vi "dbc Initial.vi"(8 "error in (no error)":errorcluster) -> (0 "error out":errorcluster, 2 "NameShort":string[][](array[string])=[["Radar_AK_AMP", "Radar_AK_ANG", "Radar_AK_BSD_FLG", "Radar_AK_DST", "Radar_AK_ELE", "Radar_AK_EXST_PRB", "Radar_AK_Ego_Car_SPD", "Radar_AK_ID", "Radar_AK_LNG_ACC", "Radar_AK_MOV_FLG", "Radar_AK_RESERVE", "Radar_AK_SPD", "Radar_AK_Vx", "Radar_AK_Vy", "Radar_AK_Vz", "", "", "", "", "", "", "", "", "", "", "", "", "", "", ""], ["Radar_BK_2_AMP", "Radar_BK_2_ANG", "Radar_BK_2_DST", "Radar_BK_2_ELE", "Radar_BK_2_SPD", "Radar_BK_3_AMP", "Radar_BK_3_ANG", "Radar_BK_3_DST", "Radar_BK_3_ELE", "Radar_BK_3_SPD", "Radar_BK_4_AMP", "Radar_BK_4_ANG", "Radar_BK_4_DST", "Radar_BK_4_ELE", "Radar_BK_4_SPD", "Radar_BK_5_AMP", "Radar_BK_5_ANG", "Radar_BK_5_DST", "Radar_BK_5_ELE", "Radar_BK_5_SPD", "Radar_BK_6_AMP", "Radar_BK_6_ANG", "Radar_BK_6_DST", "Radar_BK_6_ELE", "Radar_BK_6_SPD", "Radar_BK_AMP", "Radar_BK_ANG", "Radar_BK_DST", "Radar_BK_ELE", "Radar_BK_SPD"], ["Radar_Header_Cdi_Number", "Radar_Header_Frame_Peroid", "Radar_Header_Frame_Type", "Radar_Header_Frame_id", "Radar_Header_Raw_Number", "Radar_Header_Track_Output_Number", "", "", "", "", "", "", "", "", "", "", "", "", "", "", "", "", "", "", "", "", "", "", "", ""], ["Radar_AK_Header_Number", "Radar_AK_Run_Time", "", "", "", "", "", "", "", "", "", "", "", "", "", "", "", "", "", "", "", "", "", "", "", "", "", "", "", ""]], 3 "Session Out":refnum<k21>[](array[refnum]), 5 "ID":u32[](array[numeric])=[1280, 1024, 768, 816] format="%.0x")   [LabVIEW 2024]
uses:
  <vilib>/xnet/xnet.llb/XNET Create Session (Conversion).vi
  <resource>/objmgr/xnet.rc
panel:
  out "Sigs":refnum<k21>[][](array[refnum])
  out "XNET_DBC":T1(array[cluster])=[[{"NameShort"="Radar_AK_AMP", "ByteOrdr"=0, "StartBit"=64, "NumBits"=16, "Max"=327.67, "Min"=-327.68, "ScaleFac"=0.01, "ScaleOff"=0.0, "Comment"="", "Unit"="dB", "PDU"="Radar2ECU_AK_FRAME_0x500_pdu\nradar com1"}, {"NameShort"="Radar_AK_ANG", "ByteOrdr"=0, "StartBit"=16, "NumBits"=16, "Max"=327.67, "Min"=-327.68, "ScaleFac"=0.01, "ScaleOff"=0.0, "Comment"="", "Unit"="deg", "PDU"="Radar2ECU_AK_FRAME_0x500_pdu\nradar com1"}, {"NameShort"="Radar_AK_BSD_FLG", "ByteOrdr"=0, "StartBit"=192, "NumBits"=1, "Max"=1.0, "Min"=0.0, "ScaleFac"=1.0, "ScaleOff"=0.0, "Comment"="", "Unit"="", "PDU"="Radar2ECU_AK_FRAME_0x500_pdu\nradar com1"}, {"NameShort"="Radar_AK_DST", "ByteOrdr"=0, "StartBit"=48, "NumBits"=16, "Max"=327.67, "Min"=-327.68, "ScaleFac"=0.01, "ScaleOff"=0.0, "Comment"="", "Unit"="m", "PDU"="Radar2ECU_AK_FRAME_0x500_pdu\nradar com1"}, {"NameShort"="Radar_AK_ELE", "ByteOrdr"=0, "StartBit"=80, "NumBits"=16, "Max"=327.67, "Min"=-327.68, "ScaleFac"=0.01, "ScaleOff"=0.0, "Comment"="", "Unit"="deg", "PDU"="Radar2ECU_AK_FRAME_0x500_pdu\nradar com1"}, {"NameShort"="Radar_AK_EXST_PRB", "ByteOrdr"=0, "StartBit"=144, "NumBits"=16, "Max"=327.67, "Min"=-327.68, "ScaleFac"=0.01, "ScaleOff"=0.0, "Comment"="", "Unit"="%", "PDU"="Radar2ECU_AK_FRAME_0x500_pdu\nradar com1"}, {"NameShort"="Radar_AK_Ego_Car_SPD", "ByteOrdr"=0, "StartBit"=176, "NumBits"=16, "Max"=327.67, "Min"=-327.68, "ScaleFac"=0.01, "ScaleOff"=0.0, "Comment"="", "Unit"="m/s", "PDU"="Radar2ECU_AK_FRAME_0x500_pdu\nradar com1"}, {"NameShort"="Radar_AK_ID", "ByteOrdr"=0, "StartBit"=0, "NumBits"=16, "Max"=65535.0, "Min"=0.0, "ScaleFac"=1.0, "ScaleOff"=0.0, "Comment"="", "Unit"="", "PDU"="Radar2ECU_AK_FRAME_0x500_pdu\nradar com1"}, {"NameShort"="Radar_AK_LNG_ACC", "ByteOrdr"=0, "StartBit"=160, "NumBits"=16, "Max"=327.67, "Min"=-327.68, "ScaleFac"=0.01, "ScaleOff"=0.0, "Comment"="", "Unit"="m/s2", "PDU"="Radar2ECU_AK_FRAME_0x500_pdu\nradar com1"}, {"NameShort"="Radar_AK_MOV_FLG", "ByteOrdr"=0, "StartBit"=193, "NumBits"=1, "Max"=1.0, "Min"=0.0, "ScaleFac"=1.0, "ScaleOff"=0.0, "Comment"="", "Unit"="", "PDU"="Radar2ECU_AK_FRAME_0x500_pdu\nradar com1"}, {"NameShort"="Radar_AK_RESERVE", "ByteOrdr"=0, "StartBit"=194, "NumBits"=6, "Max"=63.0, "Min"=0.0, "ScaleFac"=1.0, "ScaleOff"=0.0, "Comment"="", "Unit"="", "PDU"="Radar2ECU_AK_FRAME_0x500_pdu\nradar com1"}, {"NameShort"="Radar_AK_SPD", "ByteOrdr"=0, "StartBit"=32, "NumBits"=16, "Max"=327.67, "Min"=-327.68, "ScaleFac"=0.01, "ScaleOff"=0.0, "Comment"="", "Unit"="m/s", "PDU"="Radar2ECU_AK_FRAME_0x500_pdu\nradar com1"}, {"NameShort"="Radar_AK_Vx", "ByteOrdr"=0, "StartBit"=96, "NumBits"=16, "Max"=0.0, "Min"=0.0, "ScaleFac"=0.01, "ScaleOff"=0.0, "Comment"="", "Unit"="", "PDU"="Radar2ECU_AK_FRAME_0x500_pdu\nradar com1"}, {"NameShort"="Radar_AK_Vy", "ByteOrdr"=0, "StartBit"=112, "NumBits"=16, "Max"=0.0, "Min"=0.0, "ScaleFac"=0.01, "ScaleOff"=0.0, "Comment"="", "Unit"="", "PDU"="Radar2ECU_AK_FRAME_0x500_pdu\nradar com1"}, {"NameShort"="Radar_AK_Vz", "ByteOrdr"=0, "StartBit"=128, "NumBits"=16, "Max"=0.0, "Min"=0.0, "ScaleFac"=0.01, "ScaleOff"=0.0, "Comment"="", "Unit"="", "PDU"="Radar2ECU_AK_FRAME_0x500_pdu\nradar com1"}, {"NameShort"="", "ByteOrdr"=0, "StartBit"=0, "NumBits"=0, "Max"=0.0, "Min"=0.0, "ScaleFac"=0.0, "ScaleOff"=0.0, "Comment"="", "Unit"="", "PDU"=""}, {"NameShort"="", "ByteOrdr"=0, "StartBit"=0, "NumBits"=0, "Max"=0.0, "Min"=0.0, "ScaleFac"=0.0, "ScaleOff"=0.0, "Comment"="", "Unit"="", "PDU"=""}, {"NameShort"="", "ByteOrdr"=0, "StartBit"=0, "NumBits"=0, "Max"=0.0, "Min"=0.0, "ScaleFac"=0.0, "ScaleOff"=0.0, "Comment"="", "Unit"="", "PDU"=""}, {"NameShort"="", "ByteOrdr"=0, "StartBit"=0, "NumBits"=0, "Max"=0.0, "Min"=0.0, "ScaleFac"=0.0, "ScaleOff"=0.0, "Comment"="", "Unit"="", "PDU"=""}, {"NameShort"="", "ByteOrdr"=0, "StartBit"=0, "NumBits"=0, "Max"=0.0, "Min"=0.0, "ScaleFac"=0.0, "ScaleOff"=0.0, "Comment"="", "Unit"="", "PDU"=""}, {"NameShort"="", "ByteOrdr"=0, "StartBit"=0, "NumBits"=0, "Max"=0.0, "Min"=0.0, "ScaleFac"=0.0, "ScaleOff"=0.0, "Comment"="", "Unit"="", "PDU"=""}, {"NameShort"="", "ByteOrdr"=0, "StartBit"=0, "NumBits"=0, "Max"=0.0, "Min"=0.0, "ScaleFac"=0.0, "ScaleOff"=0.0, "Comment"="", "Unit"="", "PDU"=""}, {"NameShort"="", "ByteOrdr"=0, "StartBit"=0, "NumBits"=0, "Max"=0.0, "Min"=0.0, "ScaleFac"=0.0, "ScaleOff"=0.0, "Comment"="", "Unit"="", "PDU"=""}, {"NameShort"="", "ByteOrdr"=0, "StartBit"=0, "NumBits"=0, "Max"=0.0, "Min"=0.0, "ScaleFac"=0.0, "ScaleOff"=0.0, "Comment"="", "Unit"="", "PDU"=""}, {"NameShort"="", "ByteOrdr"=0, "StartBit"=0, "NumBits"=0, "Max"=0.0, "Min"=0.0, "ScaleFac"=0.0, "ScaleOff"=0.0, "Comment"="", "Unit"="", "PDU"=""}, {"NameShort"="", "ByteOrdr"=0, "StartBit"=0, "NumBits"=0, "Max"=0.0, "Min"=0.0, "ScaleFac"=0.0, "ScaleOff"=0.0, "Comment"="", "Unit"="", "PDU"=""}, {"NameShort"="", "ByteOrdr"=0, "StartBit"=0, "NumBits"=0, "Max"=0.0, "Min"=0.0, "ScaleFac"=0.0, "ScaleOff"=0.0, "Comment"="", "Unit"="", "PDU"=""}, {"NameShort"="", "ByteOrdr"=0, "StartBit"=0, "NumBits"=0, "Max"=0.0, "Min"=0.0, "ScaleFac"=0.0, "ScaleOff"=0.0, "Comment"="", "Unit"="", "PDU"=""}, {"NameShort"="", "ByteOrdr"=0, "StartBit"=0, "NumBits"=0, "Max"=0.0, "Min"=0.0, "ScaleFac"=0.0, "ScaleOff"=0.0, "Comment"="", "Unit"="", "PDU"=""}, {"NameShort"="", "ByteOrdr"=0, "StartBit"=0, "NumBits"=0, "Max"=0.0, "Min"=0.0, "ScaleFac"=0.0, "ScaleOff"=0.0, "Comment"="", "Unit"="", "PDU"=""}], [{"NameShort"="Radar_BK_2_AMP", "ByteOrdr"=0, "StartBit"=128, "NumBits"=16, "Max"=327.67, "Min"=-327.68, "ScaleFac"=0.01, "ScaleOff"=0.0, "Comment"="", "Unit"="dB", "PDU"="Radar2ECU_BK_FRAME_0x400_pdu\nradar com1"}, {"NameShort"="Radar_BK_2_ANG", "ByteOrdr"=0, "StartBit"=80, "NumBits"=16, "Max"=327.67, "Min"=-327.68, "ScaleFac"=0.01, "ScaleOff"=0.0, "Comment"="", "Unit"="deg", "PDU"="Radar2ECU_BK_FRAME_0x400_pdu\nradar com1"}, {"NameShort"="Radar_BK_2_DST", "ByteOrdr"=0, "StartBit"=112, "NumBits"=16, "Max"=327.67, "Min"=-327.68, "ScaleFac"=0.01, "ScaleOff"=0.0, "Comment"="", "Unit"="m", "PDU"="Radar2ECU_BK_FRAME_0x400_pdu\nradar com1"}, {"NameShort"="Radar_BK_2_ELE", "ByteOrdr"=0, "StartBit"=144, "NumBits"=16, "Max"=327.67, "Min"=-327.68, "ScaleFac"=0.01, "ScaleOff"=0.0, "Comment"="", "Unit"="deg", "PDU"="Radar2ECU_BK_FRAME_0x400_pdu\nradar com1"}, {"NameShort"="Radar_BK_2_SPD", "ByteOrdr"=0, "StartBit"=96, "NumBits"=16, "Max"=327.67, "Min"=-327.68, "ScaleFac"=0.01, "ScaleOff"=0.0, "Comment"="", "Unit"="m/s", "PDU"="Radar2ECU_BK_FRAME_0x400_pdu\nradar com1"}, {"NameShort"="Radar_BK_3_AMP", "ByteOrdr"=0, "StartBit"=208, "NumBits"=16, "Max"=327.67, "Min"=-327.68, "ScaleFac"=0.01, "ScaleOff"=0.0, "Comment"="", "Unit"="dB", "PDU"="Radar2ECU_BK_FRAME_0x400_pdu\nradar com1"}, {"NameShort"="Radar_BK_3_ANG", "ByteOrdr"=0, "StartBit"=160, "NumBits"=16, "Max"=327.67, "Min"=-327.68, "ScaleFac"=0.01, "ScaleOff"=0.0, "Comment"="", "Unit"="deg", "PDU"="Radar2ECU_BK_FRAME_0x400_pdu\nradar com1"}, {"NameShort"="Radar_BK_3_DST", "ByteOrdr"=0, "StartBit"=192, "NumBits"=16, "Max"=327.67, "Min"=-327.68, "ScaleFac"=0.01, "ScaleOff"=0.0, "Comment"="", "Unit"="m", "PDU"="Radar2ECU_BK_FRAME_0x400_pdu\nradar com1"}, {"NameShort"="Radar_BK_3_ELE", "ByteOrdr"=0, "StartBit"=224, "NumBits"=16, "Max"=327.67, "Min"=-327.68, "ScaleFac"=0.01, "ScaleOff"=0.0, "Comment"="", "Unit"="deg", "PDU"="Radar2ECU_BK_FRAME_0x400_pdu\nradar com1"}, {"NameShort"="Radar_BK_3_SPD", "ByteOrdr"=0, "StartBit"=176, "NumBits"=16, "Max"=327.67, "Min"=-327.68, "ScaleFac"=0.01, "ScaleOff"=0.0, "Comment"="", "Unit"="m/s", "PDU"="Radar2ECU_BK_FRAME_0x400_pdu\nradar com1"}, {"NameShort"="Radar_BK_4_AMP", "ByteOrdr"=0, "StartBit"=288, "NumBits"=16, "Max"=327.67, "Min"=-327.68, "ScaleFac"=0.01, "ScaleOff"=0.0, "Comment"="", "Unit"="dB", "PDU"="Radar2ECU_BK_FRAME_0x400_pdu\nradar com1"}, {"NameShort"="Radar_BK_4_ANG", "ByteOrdr"=0, "StartBit"=240, "NumBits"=16, "Max"=327.67, "Min"=-327.68, "ScaleFac"=0.01, "ScaleOff"=0.0, "Comment"="", "Unit"="deg", "PDU"="Radar2ECU_BK_FRAME_0x400_pdu\nradar com1"}, {"NameShort"="Radar_BK_4_DST", "ByteOrdr"=0, "StartBit"=272, "NumBits"=16, "Max"=327.67, "Min"=-327.68, "ScaleFac"=0.01, "ScaleOff"=0.0, "Comment"="", "Unit"="m", "PDU"="Radar2ECU_BK_FRAME_0x400_pdu\nradar com1"}, {"NameShort"="Radar_BK_4_ELE", "ByteOrdr"=0, "StartBit"=304, "NumBits"=16, "Max"=327.67, "Min"=-327.68, "ScaleFac"=0.01, "ScaleOff"=0.0, "Comment"="", "Unit"="deg", "PDU"="Radar2ECU_BK_FRAME_0x400_pdu\nradar com1"}, {"NameShort"="Radar_BK_4_SPD", "ByteOrdr"=0, "StartBit"=256, "NumBits"=16, "Max"=327.67, "Min"=-327.68, "ScaleFac"=0.01, "ScaleOff"=0.0, "Comment"="", "Unit"="m/s", "PDU"="Radar2ECU_BK_FRAME_0x400_pdu\nradar com1"}, {"NameShort"="Radar_BK_5_AMP", "ByteOrdr"=0, "StartBit"=368, "NumBits"=16, "Max"=327.67, "Min"=-327.68, "ScaleFac"=0.01, "ScaleOff"=0.0, "Comment"="", "Unit"="dB", "PDU"="Radar2ECU_BK_FRAME_0x400_pdu\nradar com1"}, {"NameShort"="Radar_BK_5_ANG", "ByteOrdr"=0, "StartBit"=320, "NumBits"=16, "Max"=327.67, "Min"=-327.68, "ScaleFac"=0.01, "ScaleOff"=0.0, "Comment"="", "Unit"="deg", "PDU"="Radar2ECU_BK_FRAME_0x400_pdu\nradar com1"}, {"NameShort"="Radar_BK_5_DST", "ByteOrdr"=0, "StartBit"=352, "NumBits"=16, "Max"=327.67, "Min"=-327.68, "ScaleFac"=0.01, "ScaleOff"=0.0, "Comment"="", "Unit"="m", "PDU"="Radar2ECU_BK_FRAME_0x400_pdu\nradar com1"}, {"NameShort"="Radar_BK_5_ELE", "ByteOrdr"=0, "StartBit"=384, "NumBits"=16, "Max"=327.67, "Min"=-327.68, "ScaleFac"=0.01, "ScaleOff"=0.0, "Comment"="", "Unit"="deg", "PDU"="Radar2ECU_BK_FRAME_0x400_pdu\nradar com1"}, {"NameShort"="Radar_BK_5_SPD", "ByteOrdr"=0, "StartBit"=336, "NumBits"=16, "Max"=327.67, "Min"=-327.68, "ScaleFac"=0.01, "ScaleOff"=0.0, "Comment"="", "Unit"="m/s", "PDU"="Radar2ECU_BK_FRAME_0x400_pdu\nradar com1"}, {"NameShort"="Radar_BK_6_AMP", "ByteOrdr"=0, "StartBit"=448, "NumBits"=16, "Max"=327.67, "Min"=-327.68, "ScaleFac"=0.01, "ScaleOff"=0.0, "Comment"="", "Unit"="dB", "PDU"="Radar2ECU_BK_FRAME_0x400_pdu\nradar com1"}, {"NameShort"="Radar_BK_6_ANG", "ByteOrdr"=0, "StartBit"=400, "NumBits"=16, "Max"=327.67, "Min"=-327.68, "ScaleFac"=0.01, "ScaleOff"=0.0, "Comment"="", "Unit"="deg", "PDU"="Radar2ECU_BK_FRAME_0x400_pdu\nradar com1"}, {"NameShort"="Radar_BK_6_DST", "ByteOrdr"=0, "StartBit"=432, "NumBits"=16, "Max"=327.67, "Min"=-327.68, "ScaleFac"=0.01, "ScaleOff"=0.0, "Comment"="", "Unit"="m", "PDU"="Radar2ECU_BK_FRAME_0x400_pdu\nradar com1"}, {"NameShort"="Radar_BK_6_ELE", "ByteOrdr"=0, "StartBit"=464, "NumBits"=16, "Max"=327.67, "Min"=-327.68, "ScaleFac"=0.01, "ScaleOff"=0.0, "Comment"="", "Unit"="deg", "PDU"="Radar2ECU_BK_FRAME_0x400_pdu\nradar com1"}, {"NameShort"="Radar_BK_6_SPD", "ByteOrdr"=0, "StartBit"=416, "NumBits"=16, "Max"=327.67, "Min"=-327.68, "ScaleFac"=0.01, "ScaleOff"=0.0, "Comment"="", "Unit"="m/s", "PDU"="Radar2ECU_BK_FRAME_0x400_pdu\nradar com1"}, {"NameShort"="Radar_BK_AMP", "ByteOrdr"=0, "StartBit"=48, "NumBits"=16, "Max"=327.67, "Min"=-327.68, "ScaleFac"=0.01, "ScaleOff"=0.0, "Comment"="", "Unit"="dB", "PDU"="Radar2ECU_BK_FRAME_0x400_pdu\nradar com1"}, {"NameShort"="Radar_BK_ANG", "ByteOrdr"=0, "StartBit"=0, "NumBits"=16, "Max"=327.67, "Min"=-327.68, "ScaleFac"=0.01, "ScaleOff"=0.0, "Comment"="", "Unit"="deg", "PDU"="Radar2ECU_BK_FRAME_0x400_pdu\nradar com1"}, {"NameShort"="Radar_BK_DST", "ByteOrdr"=0, "StartBit"=32, "NumBits"=16, "Max"=327.67, "Min"=-327.68, "ScaleFac"=0.01, "ScaleOff"=0.0, "Comment"="", "Unit"="m", "PDU"="Radar2ECU_BK_FRAME_0x400_pdu\nradar com1"}, {"NameShort"="Radar_BK_ELE", "ByteOrdr"=0, "StartBit"=64, "NumBits"=16, "Max"=327.67, "Min"=-327.68, "ScaleFac"=0.01, "ScaleOff"=0.0, "Comment"="", "Unit"="deg", "PDU"="Radar2ECU_BK_FRAME_0x400_pdu\nradar com1"}, {"NameShort"="Radar_BK_SPD", "ByteOrdr"=0, "StartBit"=16, "NumBits"=16, "Max"=327.67, "Min"=-327.68, "ScaleFac"=0.01, "ScaleOff"=0.0, "Comment"="", "Unit"="m/s", "PDU"="Radar2ECU_BK_FRAME_0x400_pdu\nradar com1"}], [{"NameShort"="Radar_Header_Cdi_Number", "ByteOrdr"=0, "StartBit"=80, "NumBits"=16, "Max"=1024.0, "Min"=0.0, "ScaleFac"=1.0, "ScaleOff"=0.0, "Comment"="", "Unit"="", "PDU"="Radar2ECU_HEAD_FRAME_0x300_pdu\nradar com1"}, {"NameShort"="Radar_Header_Frame_Peroid", "ByteOrdr"=0, "StartBit"=0, "NumBits"=16, "Max"=655.35, "Min"=0.0, "ScaleFac"=0.01, "ScaleOff"=0.0, "Comment"="", "Unit"="ms", "PDU"="Radar2ECU_HEAD_FRAME_0x300_pdu\nradar com1"}, {"NameShort"="Radar_Header_Frame_Type", "ByteOrdr"=0, "StartBit"=16, "NumBits"=16, "Max"=7.0, "Min"=0.0, "ScaleFac"=1.0, "ScaleOff"=0.0, "Comment"="", "Unit"="", "PDU"="Radar2ECU_HEAD_FRAME_0x300_pdu\nradar com1"}, {"NameShort"="Radar_Header_Frame_id", "ByteOrdr"=0, "StartBit"=32, "NumBits"=16, "Max"=65535.0, "Min"=0.0, "ScaleFac"=1.0, "ScaleOff"=0.0, "Comment"="", "Unit"="", "PDU"="Radar2ECU_HEAD_FRAME_0x300_pdu\nradar com1"}, {"NameShort"="Radar_Header_Raw_Number", "ByteOrdr"=0, "StartBit"=48, "NumBits"=16, "Max"=1024.0, "Min"=0.0, "ScaleFac"=1.0, "ScaleOff"=0.0, "Comment"="", "Unit"="", "PDU"="Radar2ECU_HEAD_FRAME_0x300_pdu\nradar com1"}, {"NameShort"="Radar_Header_Track_Output_Number", "ByteOrdr"=0, "StartBit"=64, "NumBits"=16, "Max"=1024.0, "Min"=0.0, "ScaleFac"=1.0, "ScaleOff"=0.0, "Comment"="", "Unit"="", "PDU"="Radar2ECU_HEAD_FRAME_0x300_pdu\nradar com1"}, {"NameShort"="", "ByteOrdr"=0, "StartBit"=0, "NumBits"=0, "Max"=0.0, "Min"=0.0, "ScaleFac"=0.0, "ScaleOff"=0.0, "Comment"="", "Unit"="", "PDU"=""}, {"NameShort"="", "ByteOrdr"=0, "StartBit"=0, "NumBits"=0, "Max"=0.0, "Min"=0.0, "ScaleFac"=0.0, "ScaleOff"=0.0, "Comment"="", "Unit"="", "PDU"=""}, {"NameShort"="", "ByteOrdr"=0, "StartBit"=0, "NumBits"=0, "Max"=0.0, "Min"=0.0, "ScaleFac"=0.0, "ScaleOff"=0.0, "Comment"="", "Unit"="", "PDU"=""}, {"NameShort"="", "ByteOrdr"=0, "StartBit"=0, "NumBits"=0, "Max"=0.0, "Min"=0.0, "ScaleFac"=0.0, "ScaleOff"=0.0, "Comment"="", "Unit"="", "PDU"=""}, {"NameShort"="", "ByteOrdr"=0, "StartBit"=0, "NumBits"=0, "Max"=0.0, "Min"=0.0, "ScaleFac"=0.0, "ScaleOff"=0.0, "Comment"="", "Unit"="", "PDU"=""}, {"NameShort"="", "ByteOrdr"=0, "StartBit"=0, "NumBits"=0, "Max"=0.0, "Min"=0.0, "ScaleFac"=0.0, "ScaleOff"=0.0, "Comment"="", "Unit"="", "PDU"=""}, {"NameShort"="", "ByteOrdr"=0, "StartBit"=0, "NumBits"=0, "Max"=0.0, "Min"=0.0, "ScaleFac"=0.0, "ScaleOff"=0.0, "Comment"="", "Unit"="", "PDU"=""}, {"NameShort"="", "ByteOrdr"=0, "StartBit"=0, "NumBits"=0, "Max"=0.0, "Min"=0.0, "ScaleFac"=0.0, "ScaleOff"=0.0, "Comment"="", "Unit"="", "PDU"=""}, {"NameShort"="", "ByteOrdr"=0, "StartBit"=0, "NumBits"=0, "Max"=0.0, "Min"=0.0, "ScaleFac"=0.0, "ScaleOff"=0.0, "Comment"="", "Unit"="", "PDU"=""}, {"NameShort"="", "ByteOrdr"=0, "StartBit"=0, "NumBits"=0, "Max"=0.0, "Min"=0.0, "ScaleFac"=0.0, "ScaleOff"=0.0, "Comment"="", "Unit"="", "PDU"=""}, {"NameShort"="", "ByteOrdr"=0, "StartBit"=0, "NumBits"=0, "Max"=0.0, "Min"=0.0, "ScaleFac"=0.0, "ScaleOff"=0.0, "Comment"="", "Unit"="", "PDU"=""}, {"NameShort"="", "ByteOrdr"=0, "StartBit"=0, "NumBits"=0, "Max"=0.0, "Min"=0.0, "ScaleFac"=0.0, "ScaleOff"=0.0, "Comment"="", "Unit"="", "PDU"=""}, {"NameShort"="", "ByteOrdr"=0, "StartBit"=0, "NumBits"=0, "Max"=0.0, "Min"=0.0, "ScaleFac"=0.0, "ScaleOff"=0.0, "Comment"="", "Unit"="", "PDU"=""}, {"NameShort"="", "ByteOrdr"=0, "StartBit"=0, "NumBits"=0, "Max"=0.0, "Min"=0.0, "ScaleFac"=0.0, "ScaleOff"=0.0, "Comment"="", "Unit"="", "PDU"=""}, {"NameShort"="", "ByteOrdr"=0, "StartBit"=0, "NumBits"=0, "Max"=0.0, "Min"=0.0, "ScaleFac"=0.0, "ScaleOff"=0.0, "Comment"="", "Unit"="", "PDU"=""}, {"NameShort"="", "ByteOrdr"=0, "StartBit"=0, "NumBits"=0, "Max"=0.0, "Min"=0.0, "ScaleFac"=0.0, "ScaleOff"=0.0, "Comment"="", "Unit"="", "PDU"=""}, {"NameShort"="", "ByteOrdr"=0, "StartBit"=0, "NumBits"=0, "Max"=0.0, "Min"=0.0, "ScaleFac"=0.0, "ScaleOff"=0.0, "Comment"="", "Unit"="", "PDU"=""}, {"NameShort"="", "ByteOrdr"=0, "StartBit"=0, "NumBits"=0, "Max"=0.0, "Min"=0.0, "ScaleFac"=0.0, "ScaleOff"=0.0, "Comment"="", "Unit"="", "PDU"=""}, {"NameShort"="", "ByteOrdr"=0, "StartBit"=0, "NumBits"=0, "Max"=0.0, "Min"=0.0, "ScaleFac"=0.0, "ScaleOff"=0.0, "Comment"="", "Unit"="", "PDU"=""}, {"NameShort"="", "ByteOrdr"=0, "StartBit"=0, "NumBits"=0, "Max"=0.0, "Min"=0.0, "ScaleFac"=0.0, "ScaleOff"=0.0, "Comment"="", "Unit"="", "PDU"=""}, {"NameShort"="", "ByteOrdr"=0, "StartBit"=0, "NumBits"=0, "Max"=0.0, "Min"=0.0, "ScaleFac"=0.0, "ScaleOff"=0.0, "Comment"="", "Unit"="", "PDU"=""}, {"NameShort"="", "ByteOrdr"=0, "StartBit"=0, "NumBits"=0, "Max"=0.0, "Min"=0.0, "ScaleFac"=0.0, "ScaleOff"=0.0, "Comment"="", "Unit"="", "PDU"=""}, {"NameShort"="", "ByteOrdr"=0, "StartBit"=0, "NumBits"=0, "Max"=0.0, "Min"=0.0, "ScaleFac"=0.0, "ScaleOff"=0.0, "Comment"="", "Unit"="", "PDU"=""}, {"NameShort"="", "ByteOrdr"=0, "StartBit"=0, "NumBits"=0, "Max"=0.0, "Min"=0.0, "ScaleFac"=0.0, "ScaleOff"=0.0, "Comment"="", "Unit"="", "PDU"=""}], [{"NameShort"="Radar_AK_Header_Number", "ByteOrdr"=0, "StartBit"=0, "NumBits"=16, "Max"=0.0, "Min"=0.0, "ScaleFac"=1.0, "ScaleOff"=0.0, "Comment"="", "Unit"="", "PDU"="Radar2ECU_HEAD_FRAME_0x330_pdu\nradar com1"}, {"NameShort"="Radar_AK_Run_Time", "ByteOrdr"=0, "StartBit"=16, "NumBits"=32, "Max"=0.0, "Min"=0.0, "ScaleFac"=1.0, "ScaleOff"=0.0, "Comment"="", "Unit"="ms", "PDU"="Radar2ECU_HEAD_FRAME_0x330_pdu\nradar com1"}, {"NameShort"="", "ByteOrdr"=0, "StartBit"=0, "NumBits"=0, "Max"=0.0, "Min"=0.0, "ScaleFac"=0.0, "ScaleOff"=0.0, "Comment"="", "Unit"="", "PDU"=""}, {"NameShort"="", "ByteOrdr"=0, "StartBit"=0, "NumBits"=0, "Max"=0.0, "Min"=0.0, "ScaleFac"=0.0, "ScaleOff"=0.0, "Comment"="", "Unit"="", "PDU"=""}, {"NameShort"="", "ByteOrdr"=0, "StartBit"=0, "NumBits"=0, "Max"=0.0, "Min"=0.0, "ScaleFac"=0.0, "ScaleOff"=0.0, "Comment"="", "Unit"="", "PDU"=""}, {"NameShort"="", "ByteOrdr"=0, "StartBit"=0, "NumBits"=0, "Max"=0.0, "Min"=0.0, "ScaleFac"=0.0, "ScaleOff"=0.0, "Comment"="", "Unit"="", "PDU"=""}, {"NameShort"="", "ByteOrdr"=0, "StartBit"=0, "NumBits"=0, "Max"=0.0, "Min"=0.0, "ScaleFac"=0.0, "ScaleOff"=0.0, "Comment"="", "Unit"="", "PDU"=""}, {"NameShort"="", "ByteOrdr"=0, "StartBit"=0, "NumBits"=0, "Max"=0.0, "Min"=0.0, "ScaleFac"=0.0, "ScaleOff"=0.0, "Comment"="", "Unit"="", "PDU"=""}, {"NameShort"="", "ByteOrdr"=0, "StartBit"=0, "NumBits"=0, "Max"=0.0, "Min"=0.0, "ScaleFac"=0.0, "ScaleOff"=0.0, "Comment"="", "Unit"="", "PDU"=""}, {"NameShort"="", "ByteOrdr"=0, "StartBit"=0, "NumBits"=0, "Max"=0.0, "Min"=0.0, "ScaleFac"=0.0, "ScaleOff"=0.0, "Comment"="", "Unit"="", "PDU"=""}, {"NameShort"="", "ByteOrdr"=0, "StartBit"=0, "NumBits"=0, "Max"=0.0, "Min"=0.0, "ScaleFac"=0.0, "ScaleOff"=0.0, "Comment"="", "Unit"="", "PDU"=""}, {"NameShort"="", "ByteOrdr"=0, "StartBit"=0, "NumBits"=0, "Max"=0.0, "Min"=0.0, "ScaleFac"=0.0, "ScaleOff"=0.0, "Comment"="", "Unit"="", "PDU"=""}, {"NameShort"="", "ByteOrdr"=0, "StartBit"=0, "NumBits"=0, "Max"=0.0, "Min"=0.0, "ScaleFac"=0.0, "ScaleOff"=0.0, "Comment"="", "Unit"="", "PDU"=""}, {"NameShort"="", "ByteOrdr"=0, "StartBit"=0, "NumBits"=0, "Max"=0.0, "Min"=0.0, "ScaleFac"=0.0, "ScaleOff"=0.0, "Comment"="", "Unit"="", "PDU"=""}, {"NameShort"="", "ByteOrdr"=0, "StartBit"=0, "NumBits"=0, "Max"=0.0, "Min"=0.0, "ScaleFac"=0.0, "ScaleOff"=0.0, "Comment"="", "Unit"="", "PDU"=""}, {"NameShort"="", "ByteOrdr"=0, "StartBit"=0, "NumBits"=0, "Max"=0.0, "Min"=0.0, "ScaleFac"=0.0, "ScaleOff"=0.0, "Comment"="", "Unit"="", "PDU"=""}, {"NameShort"="", "ByteOrdr"=0, "StartBit"=0, "NumBits"=0, "Max"=0.0, "Min"=0.0, "ScaleFac"=0.0, "ScaleOff"=0.0, "Comment"="", "Unit"="", "PDU"=""}, {"NameShort"="", "ByteOrdr"=0, "StartBit"=0, "NumBits"=0, "Max"=0.0, "Min"=0.0, "ScaleFac"=0.0, "ScaleOff"=0.0, "Comment"="", "Unit"="", "PDU"=""}, {"NameShort"="", "ByteOrdr"=0, "StartBit"=0, "NumBits"=0, "Max"=0.0, "Min"=0.0, "ScaleFac"=0.0, "ScaleOff"=0.0, "Comment"="", "Unit"="", "PDU"=""}, {"NameShort"="", "ByteOrdr"=0, "StartBit"=0, "NumBits"=0, "Max"=0.0, "Min"=0.0, "ScaleFac"=0.0, "ScaleOff"=0.0, "Comment"="", "Unit"="", "PDU"=""}, {"NameShort"="", "ByteOrdr"=0, "StartBit"=0, "NumBits"=0, "Max"=0.0, "Min"=0.0, "ScaleFac"=0.0, "ScaleOff"=0.0, "Comment"="", "Unit"="", "PDU"=""}, {"NameShort"="", "ByteOrdr"=0, "StartBit"=0, "NumBits"=0, "Max"=0.0, "Min"=0.0, "ScaleFac"=0.0, "ScaleOff"=0.0, "Comment"="", "Unit"="", "PDU"=""}, {"NameShort"="", "ByteOrdr"=0, "StartBit"=0, "NumBits"=0, "Max"=0.0, "Min"=0.0, "ScaleFac"=0.0, "ScaleOff"=0.0, "Comment"="", "Unit"="", "PDU"=""}, {"NameShort"="", "ByteOrdr"=0, "StartBit"=0, "NumBits"=0, "Max"=0.0, "Min"=0.0, "ScaleFac"=0.0, "ScaleOff"=0.0, "Comment"="", "Unit"="", "PDU"=""}, {"NameShort"="", "ByteOrdr"=0, "StartBit"=0, "NumBits"=0, "Max"=0.0, "Min"=0.0, "ScaleFac"=0.0, "ScaleOff"=0.0, "Comment"="", "Unit"="", "PDU"=""}, {"NameShort"="", "ByteOrdr"=0, "StartBit"=0, "NumBits"=0, "Max"=0.0, "Min"=0.0, "ScaleFac"=0.0, "ScaleOff"=0.0, "Comment"="", "Unit"="", "PDU"=""}, {"NameShort"="", "ByteOrdr"=0, "StartBit"=0, "NumBits"=0, "Max"=0.0, "Min"=0.0, "ScaleFac"=0.0, "ScaleOff"=0.0, "Comment"="", "Unit"="", "PDU"=""}, {"NameShort"="", "ByteOrdr"=0, "StartBit"=0, "NumBits"=0, "Max"=0.0, "Min"=0.0, "ScaleFac"=0.0, "ScaleOff"=0.0, "Comment"="", "Unit"="", "PDU"=""}, {"NameShort"="", "ByteOrdr"=0, "StartBit"=0, "NumBits"=0, "Max"=0.0, "Min"=0.0, "ScaleFac"=0.0, "ScaleOff"=0.0, "Comment"="", "Unit"="", "PDU"=""}, {"NameShort"="", "ByteOrdr"=0, "StartBit"=0, "NumBits"=0, "Max"=0.0, "Min"=0.0, "ScaleFac"=0.0, "ScaleOff"=0.0, "Comment"="", "Unit"="", "PDU"=""}]]
  out "大小":i32[](array[numeric])=[4, 30]
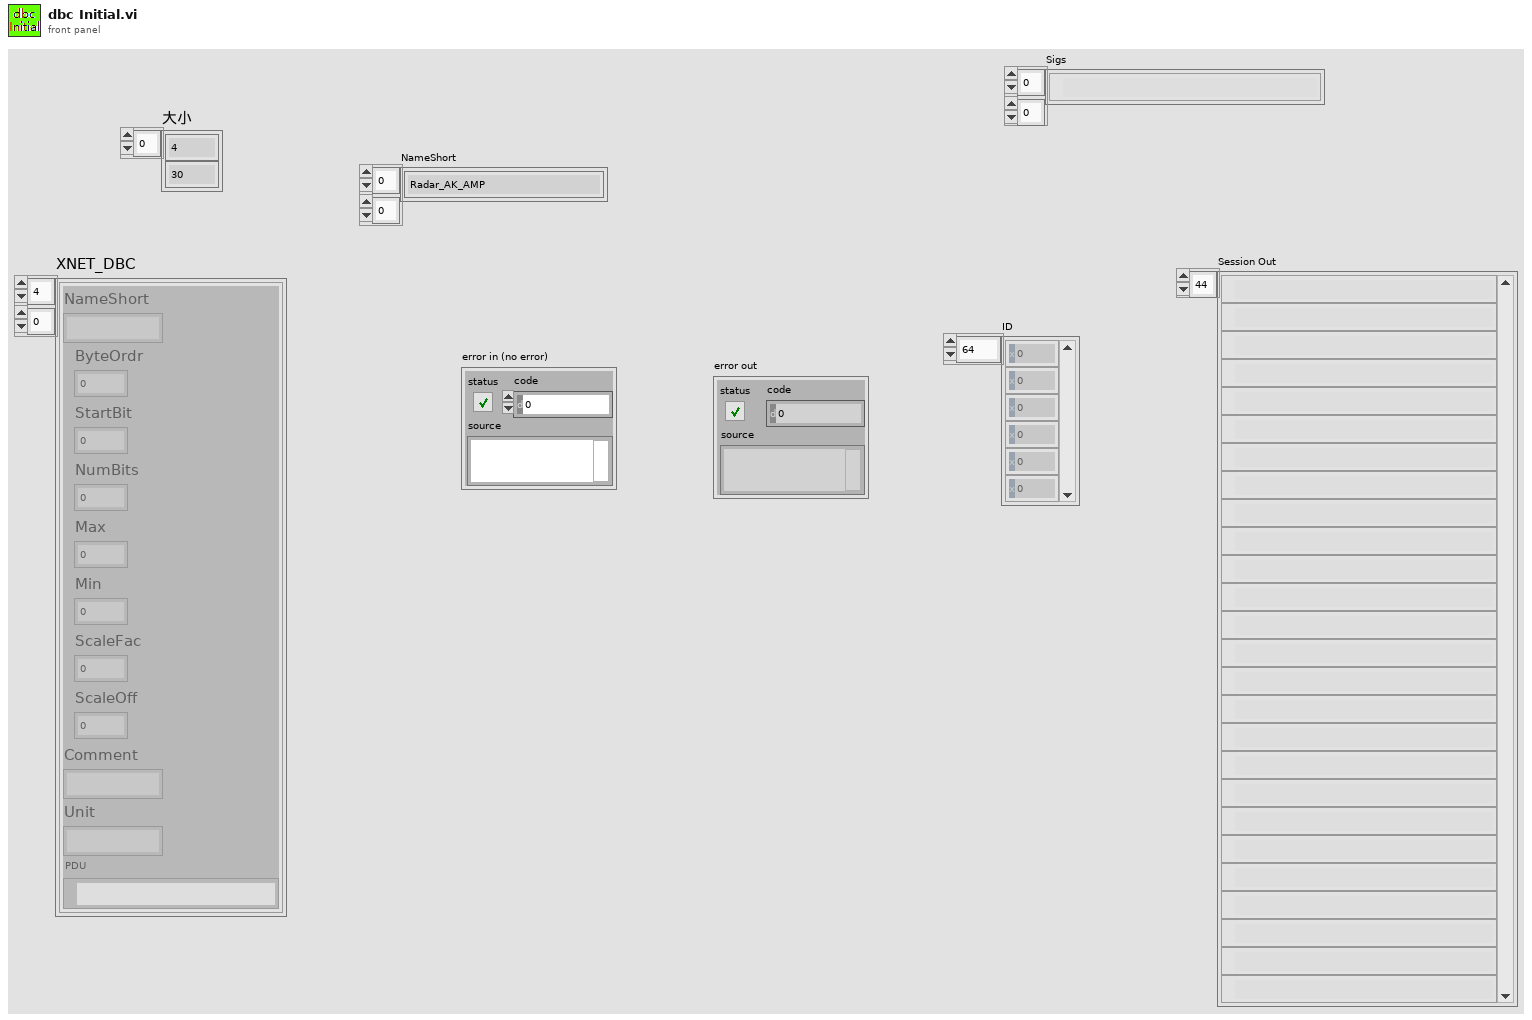
[diagram p1: front panel]
types:
  T1 = cluster{"NameShort":string, "ByteOrdr":u32, "StartBit":u32, "NumBits":u32, "Max":dbl, "Min":dbl, "ScaleFac":dbl, "ScaleOff":dbl, "Comment":string, "Unit":string, "PDU":refnum<k21>}[][]
  T2 = cluster{"NameShort":string, "ByteOrdr":u32, "StartBit":u32, "NumBits":u32, "Max":dbl, "Min":dbl, "ScaleFac":dbl, "ScaleOff":dbl, "Comment":string, "Unit":string, "PDU":refnum<k21>}
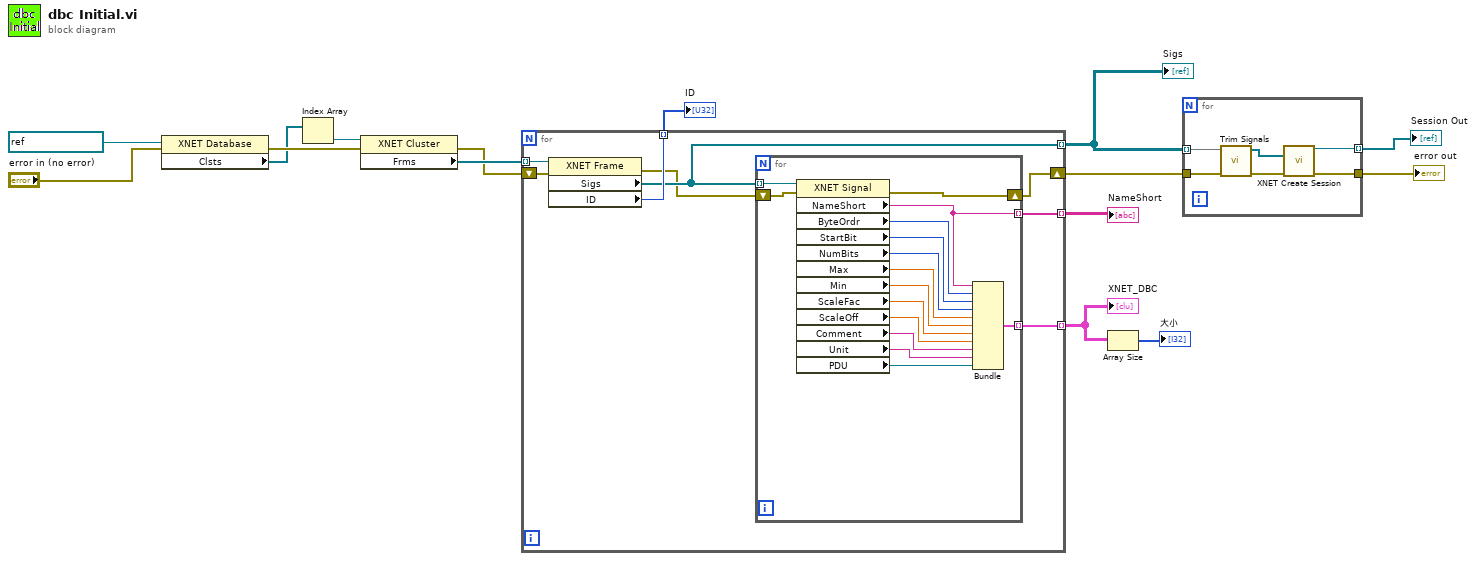
[diagram p0: block diagram]
diagram:
  n1 = property class="XNET Database"(reference=refnum<k21> "output33(1)" ("XNET Database"), error in="error in (no error)") -> (error out=w14:errorcluster, "Clsts"=w12:refnum<k21>[])  [unwired: 1 out]
  n2 = Index Array(array=w12) -> (element=w13:refnum<k21>)  [unwired: 1 in]
  n3 = property class="XNET Cluster"(reference=w13, error in=w14) -> (error out=w9:errorcluster, "Frms"=w10:refnum<k21>[])  [unwired: 1 out]
  n4 = for {
    tunnel: w10 -> [w23] mode=indexing
    tunnel: [w22] -> w7 mode=indexing
    tunnel: [w21] -> w4 mode=indexing
    tunnel: [w20] -> w3 mode=indexing
    tunnel: [w19] -> w1 mode=indexing
    shift-right: [w16] -> w6
    shift-left: w9 -> [w18]
    n5 = property class="XNET Frame"(reference=w23, error in=w18) -> (error out=w17:errorcluster, "Sigs"=w19:refnum<k21>[], "ID"=w21:u32)  [unwired: 1 out]
    n6 = for {
      tunnel: w19 -> [w38] mode=indexing
      tunnel: [w28] -> w22 mode=indexing
      tunnel: [w26] -> w20 mode=indexing
      shift-right: [w24] -> w16
      shift-left: w17 -> [w25]
      n7 = property class="XNET Signal"(reference=w38, error in=w25) -> (error out=w24:errorcluster, "NameShort"=w26:string, "ByteOrdr"=w37:u32, "StartBit"=w36:u32, "NumBits"=w35:u32, "Max"=w34:dbl, "Min"=w33:dbl, "ScaleFac"=w32:dbl, "ScaleOff"=w31:dbl, "Comment"=w30:string, "Unit"=w29:string, "PDU"=w27:refnum<k21>)  [unwired: 1 out]
      n8 = Bundle("NameShort"=w26, "ByteOrdr"=w37, "StartBit"=w36, "NumBits"=w35, "Max"=w34, "Min"=w33, "ScaleFac"=w32, "ScaleOff"=w31, "Comment"=w30, "Unit"=w29, "PDU"=w27) -> (w28:T2)  [unwired: 1 in]
    }
  }
  "XNET_DBC" <- w7
  "ID" <- w4
  "NameShort" <- w3
  "Sigs" <- w1
  n9 = Array Size(array=w7) -> (size(s)=→"大小":i32[])
  n10 = for {
    tunnel: w1 -> [w44] mode=indexing
    tunnel: [w39] -> w2 mode=indexing
    tunnel: w6 -> [w42]
    tunnel: [w40] -> w5
    n11 = call "Trim Signals.vi"("error in (no error)"=w42, "Signal In"=w44) -> ("error out (no error) 2"=w41:errorcluster, "Signal Out"=w43:refnum<k21>[])  [unwired: 8 in]
    n12 = call-poly <vilib>:"XNET Create Session.vi"("signal list"=w43, "error in (no error)"=w41) -> ("session out"=w39:refnum<k21>, "error out"=w40:errorcluster)  [unwired: 12 in]
  }
  "error out" <- w5
  "Session Out" <- w2
